vi "MetadataFromRD.vi"(10 "ChannelName":string, 11 "Raw data file":path) -> (2 "ValueString":string)   [LabVIEW 2011]
panel:
  out "Name-Value Array":string[][](array[string])
  out "index of element":i32
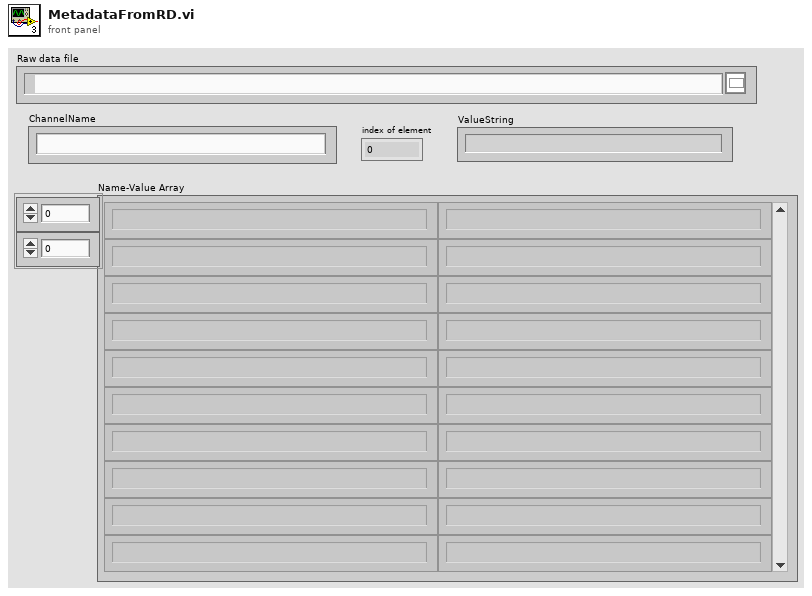
[diagram p1: front panel]
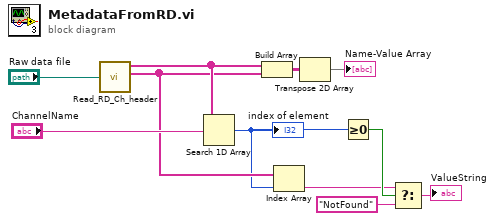
[diagram p0: block diagram]
diagram:
  n1 = call "Read_RD_Ch_header.vi"("Raw data file"="Raw data file") -> ("Ch Name Out"=w9:string[], "Ch Values"=w8:string[])  [unwired: 2 out]
  n2 = Search 1D Array(1D array=w9, element="ChannelName") -> (index of element=w5:i32)  [unwired: 1 in]
  "index of element" <- w5
  n3 = Build Array(w9, w8) -> (w7:string[][])
  n4 = Index Array(array=w8, index=w5) -> (element=w2:string)
  n5 = Transpose 2D Array(2D array=w7) -> (transposed array=→"Name-Value Array":string[][])
  n6 = Greater Or Equal To 0?(x=w5) -> (x >= 0?=w3:bool)
  n7 = Select(t=w2, s=w3, f="NotFound") -> (s? t:f=→"ValueString":string)
